vi "AssertVIFPState_Tests.vi"(8 "Error In":errorcluster) -> (0 "Error Out":errorcluster)   [LabVIEW 2016, in "DronaTest.lvlib"]
uses:
  DronaTest.lvlib
  APIs/Stimulus/KeyBoardSimulation/typedef/VirtualKey.ctl
  APIs/Stimulus/KeyBoardSimulation/typedef/Action.ctl
  APIs/Stimulus/VI/MakeVIFrontMost.vi
  APIs/Stimulus/KeyBoardSimulation/KeyboardSimulationCore.vi
  APIs/Assert/AssertVI/FPState/AssertVIFPStateMaximized.vi
  APIs/Assert/AssertVI/FPState/AssertVIFPStateStandard.vi
  APIs/Assert/AssertVI/FPState/AssertVIFPStateMinimized.vi
  APIs/Stimulus/VI/CloseVI.vi
  APIs/Assert/AssertVI/FPState/AssertVIFPStateInvalid.vi
  APIs/Assert/AssertVI/FPState/AssertVIFPStateClosed.vi
  <vilib>/addons/_JKI Toolkits/Caraya/classes/Test/Test.lvclass
  Drona.lvlib
  APIs/Stimulus/KeyBoardSimulation/KeyboardSimulation.lvlib
  <vilib>/addons/_JKI Toolkits/Caraya/classes/Assert/Assert.lvclass
  APIs/Stimulus/VI/VI.lvlib
  APIs/Assert/AssertVI/AssertVI.lvlib
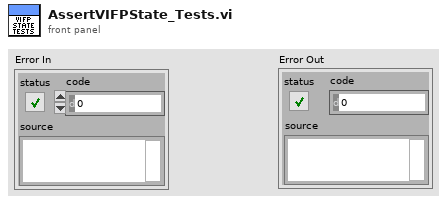
[diagram p1: front panel]
types:
  T1 = enum32{"Invalid", "Standard", "Closed", "Hidden", "Minimized", "Maximized"}
  T2 = typedef "Drona.lvlib/KeyboardSimulation.lvlib/VirtualKey.ctl" = u8
  T3 = typedef "Drona.lvlib/KeyboardSimulation.lvlib/Action.ctl" = enum16{"Press", "Up", "Down"}
  T4 = cluster{"Key":T2, "Action":T3, "Delay (ms)":u32}[]
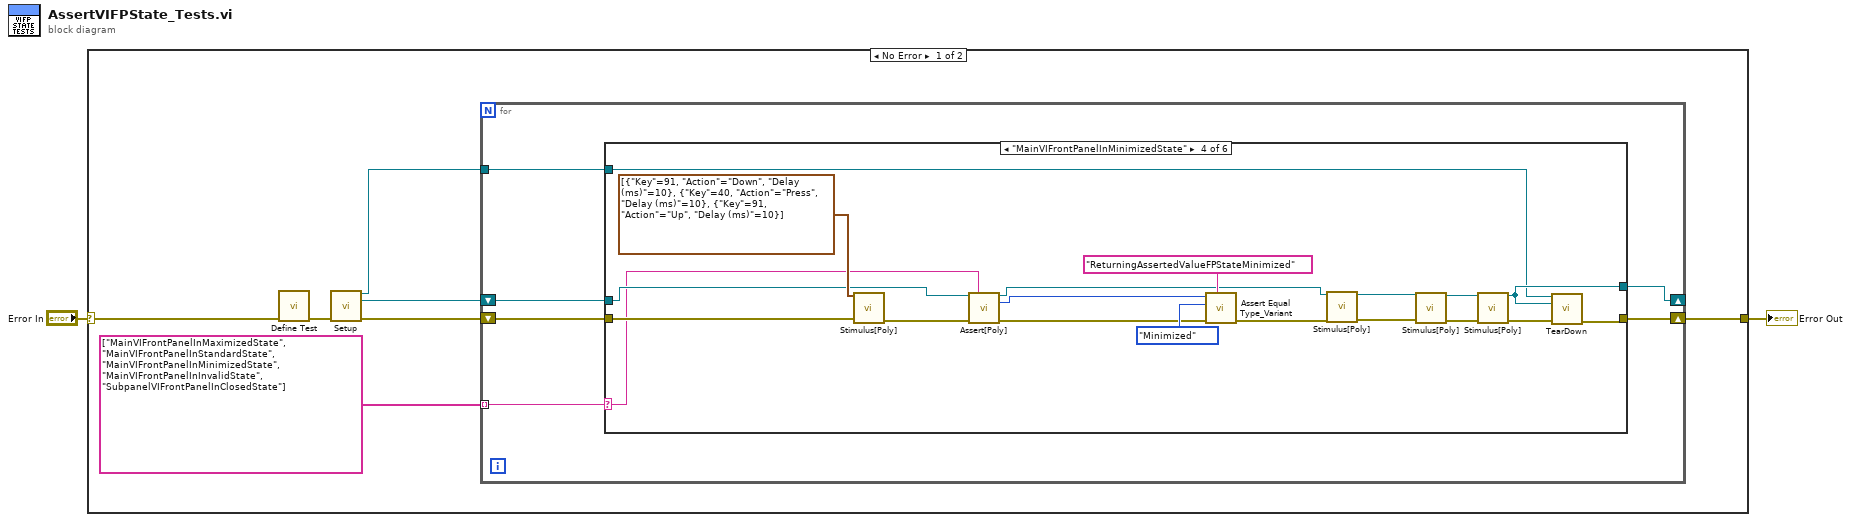
[diagram p0: block diagram]
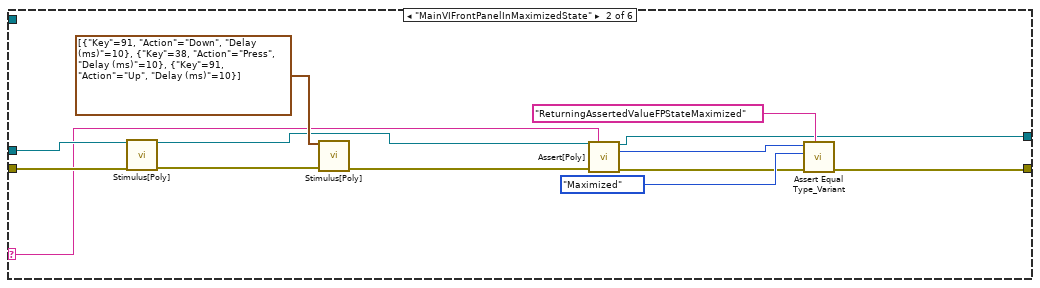
[diagram p3: hidden frame]
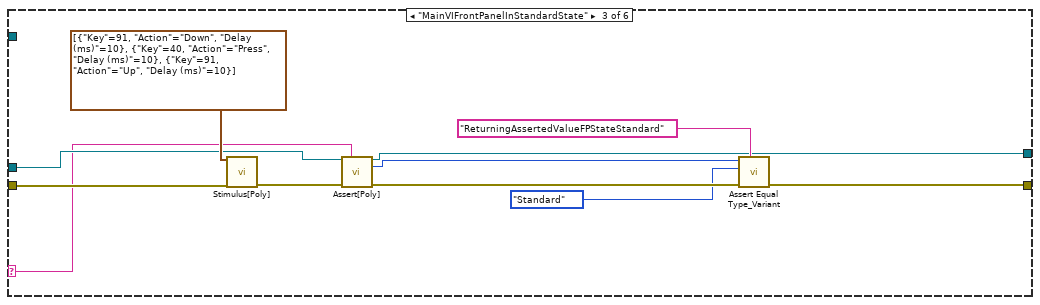
[diagram p4: hidden frame]
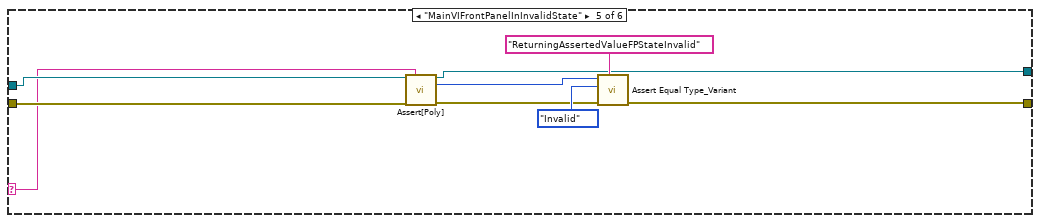
[diagram p5: hidden frame]
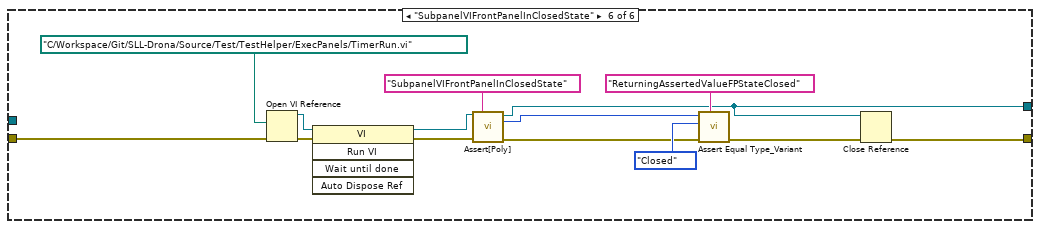
[diagram p6: hidden frame]
diagram:
  n1 = case shown="No Error" "Error In" {
    selector: "Error In" -> [w8 w84]
    tunnel: [w3 w84] -> w1
    frame No Error {
      n2 = call <vilib>:"Define Test.vi"("error in (no error)"=w8) -> ("error out"=w9:errorcluster)  [unwired: 9 in, 1 out]
      n3 = call "Setup.vi"("error in (no error)"=w9) -> ("Application Ref"=w4:refnum<vi>, "VI out"=w5:refnum<vi>, "error out"=w6:errorcluster)  [unwired: 12 in]
      n4 = for {
        tunnel: string[] ["MainVIFrontPanelInMaximizedState", "MainVIFrontPanelInStandardState", "MainVIFrontPanelInMinimizedState", "MainVIFrontPanelInInvalidState", "SubpanelVIFrontPanelInClosedState"] ("Label") -> [w15] mode=indexing
        shift-right: [w13] -> w3
        shift-left: w6 -> [w14]
        shift-right: [w11] -> _
        shift-left: w5 -> [w12]
        tunnel: w4 -> [w10]
        n5 = case shown="\"MainVIFrontPanelInMinimizedState\"" w15 {
          selector: w15 -> [_ w18 w32 w43 w61 _]
          tunnel: w14 -> [w17 w22 w36 w48 w65 w74]
          tunnel: [w17 w21 w35 w46 w64 w72] -> w13
          tunnel: w12 -> [w16 w20 w33 w44 w63 _]
          tunnel: [w16 w19 w31 w45 w62 w71] -> w11
          tunnel: w10 -> [_ _ _ w42 _ _]
          frame Default {
          }
          frame "MainVIFrontPanelInMaximizedState" {
            n6 = call-poly "Stimulus[Poly].vi"("VI Reference In"=w20, "error in"=w22) -> ("VI Reference Out"=w24:refnum<vi>, "error out"=w23:errorcluster)  [unwired: 12 in]
            n7 = call-poly "Stimulus[Poly].vi"("Key Array"=T4 [{"Key"=91, "Action"=enum."Down", "Delay (ms)"=10}, {"Key"=38, "Action"=enum."Press", "Delay (ms)"=10}, {"Key"=91, "Action"=enum."Up", "Delay (ms)"=10}], "error in"=w23) -> ("error out"=w29:errorcluster)  [unwired: 13 in]
            n8 = call-poly "Assert[Poly].vi"("VI Reference In"=w24, "Label"=w18, "Error In"=w29) -> ("VI Reference Out"=w19:refnum<vi>, "Asserted Value"=w26:T1, "Error Out"=w27:errorcluster)  [unwired: 10 in]
            n9 = call <vilib>:"Assert Equal Type_Variant.vi"("Label"="ReturningAssertedValueFPStateMaximized", "error in (no error)"=w27, "Y"=T1."Maximized" ("Asserted Value"), "X"=w26) -> ("error out"=w21:errorcluster)  [unwired: 6 in, 1 out]
          }
          frame "MainVIFrontPanelInStandardState" {
            n10 = call-poly "Stimulus[Poly].vi"("Key Array"=T4 [{"Key"=91, "Action"=enum."Down", "Delay (ms)"=10}, {"Key"=40, "Action"=enum."Press", "Delay (ms)"=10}, {"Key"=91, "Action"=enum."Up", "Delay (ms)"=10}], "error in"=w36) -> ("error out"=w37:errorcluster)  [unwired: 13 in]
            n11 = call-poly "Assert[Poly].vi"("VI Reference In"=w33, "Label"=w32, "Error In"=w37) -> ("VI Reference Out"=w31:refnum<vi>, "Asserted Value"=w40:T1, "Error Out"=w41:errorcluster)  [unwired: 10 in]
            n12 = call <vilib>:"Assert Equal Type_Variant.vi"("Label"="ReturningAssertedValueFPStateStandard", "error in (no error)"=w41, "Y"=T1."Standard" ("Asserted Value"), "X"=w40) -> ("error out"=w35:errorcluster)  [unwired: 6 in, 1 out]
          }
          frame "MainVIFrontPanelInMinimizedState" {
            n13 = call-poly "Stimulus[Poly].vi"("Key Array"=T4 [{"Key"=91, "Action"=enum."Down", "Delay (ms)"=10}, {"Key"=40, "Action"=enum."Press", "Delay (ms)"=10}, {"Key"=91, "Action"=enum."Up", "Delay (ms)"=10}], "error in"=w48) -> ("error out"=w60:errorcluster)  [unwired: 13 in]
            n14 = call-poly "Assert[Poly].vi"("VI Reference In"=w44, "Label"=w43, "Error In"=w60) -> ("VI Reference Out"=w53:refnum<vi>, "Asserted Value"=w56:T1, "Error Out"=w55:errorcluster)  [unwired: 10 in]
            n15 = call <vilib>:"Assert Equal Type_Variant.vi"("Label"="ReturningAssertedValueFPStateMinimized", "error in (no error)"=w55, "Y"=T1."Minimized" ("Asserted Value"), "X"=w56) -> ("error out"=w54:errorcluster)  [unwired: 6 in, 1 out]
            n16 = call-poly "Stimulus[Poly].vi"("VI Reference In"=w53, "error in"=w54) -> ("VI Reference Out"=w51:refnum<vi>, "error out"=w52:errorcluster)  [unwired: 12 in]
            n17 = call-poly "Stimulus[Poly].vi"("VI Reference In"=w51, "error in"=w52) -> ("VI Reference Out"=w49:refnum<vi>, "error out"=w50:errorcluster)  [unwired: 12 in]
            n18 = call-poly "Stimulus[Poly].vi"("VI Reference In"=w49, "error in"=w50) -> ("VI Reference Out"=w45:refnum<vi>, "error out"=w47:errorcluster)  [unwired: 12 in]
            n19 = call "TearDown.vi"("Application Ref"=w42, "VI in"=w45, "error in (no error)"=w47) -> ("error out"=w46:errorcluster)  [unwired: 12 in]
          }
          frame "MainVIFrontPanelInInvalidState" {
            n20 = call-poly "Assert[Poly].vi"("VI Reference In"=w63, "Label"=w61, "Error In"=w65) -> ("VI Reference Out"=w62:refnum<vi>, "Asserted Value"=w69:T1, "Error Out"=w66:errorcluster)  [unwired: 10 in]
            n21 = call <vilib>:"Assert Equal Type_Variant.vi"("Label"="ReturningAssertedValueFPStateInvalid", "error in (no error)"=w66, "Y"=T1."Invalid" ("Asserted Value"), "X"=w69) -> ("error out"=w64:errorcluster)  [unwired: 6 in, 1 out]
          }
          frame "SubpanelVIFrontPanelInClosedState" {
            n22 = Open VI Reference(vi path=path "C:/Workspace/Git/SLL-Drona/Source/Test/TestHelper/ExecPanels/TimerRun.vi", error in (no error)=w74) -> (vi reference=w83:refnum<vi>, error out=w82:errorcluster)  [unwired: 4 in]
            n23 = invoke class="VI" method="Run VI"(reference=w83, error in=w82) -> (reference out=w77:refnum<vi>, error out=w78:errorcluster)  [unwired: 3 in, 3 out]
            n24 = call-poly "Assert[Poly].vi"("VI Reference In"=w77, "Label"="SubpanelVIFrontPanelInClosedState", "Error In"=w78) -> ("VI Reference Out"=w71:refnum<vi>, "Asserted Value"=w79:T1, "Error Out"=w76:errorcluster)  [unwired: 10 in]
            n25 = call <vilib>:"Assert Equal Type_Variant.vi"("Label"="ReturningAssertedValueFPStateClosed", "error in (no error)"=w76, "Y"=T1."Closed" ("Asserted Value"), "X"=w79) -> ("error out"=w73:errorcluster)  [unwired: 6 in, 1 out]
            n26 = Close Reference(reference=w71, error in (no error)=w73) -> (error out=w72:errorcluster)
          }
        }
      }
    }
    frame Error {
    }
  }
  "Error Out" <- w1
